vi "Save Macro.vi"(7 "Macro Name":string, 8 "error in (no error)":errorcluster, 10 "Macro Cluster":T1, 11 "refnum":T4) -> (0 "error out":errorcluster, 3 "refnum out":T4)   [LabVIEW 2023]
doc: "Saves <B>Macro Cluster</B> and its associated <B>Macro Name</B> to the config file defined by <B>refnum</B>."
uses:
  <vilib>/Utility/config.llb/Config Data RefNum.ctl
  CTLs/Macro Cluster V3.ctl
  CTLs/Step V3.ctl
  CTLs/Step Type V3.ctl
  <vilib>/Utility/config.llb/Write Key (String).vi
  <vilib>/Utility/config.llb/Write Key (I32).vi
  <vilib>/Utility/config.llb/NI_LVConfig.lvlib
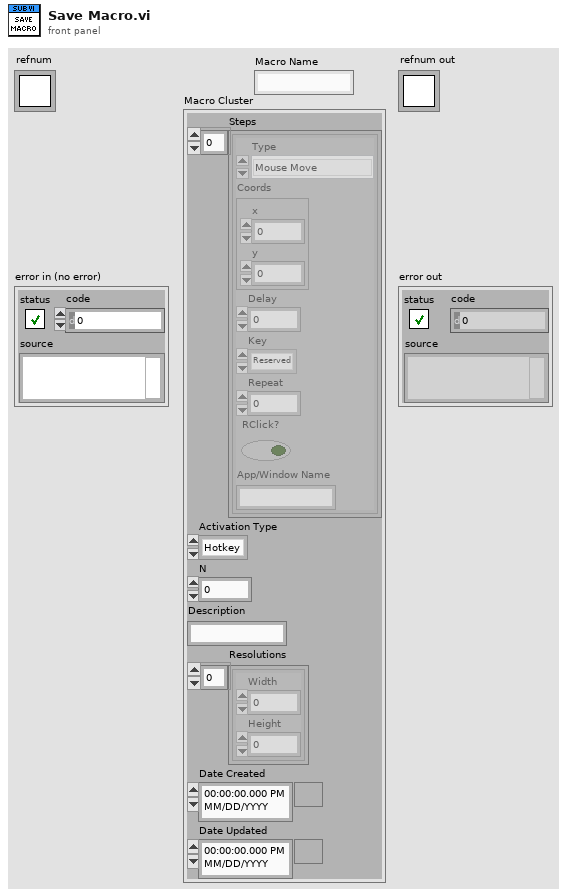
[diagram p1: front panel]
types:
  T1 = typedef "Macro Cluster V3.ctl" = cluster{"Steps":T2[], "Activation Type":enum32{"Hotkey", "Automatic"}, "N":i32, "Description":string, "Resolutions":cluster{"Width":i16, "Height":i16}[], "Date Created":timestamp, "Date Updated":timestamp}
  T2 = typedef "Step V3.ctl" = cluster{"Type":T3, "Coords":cluster{"x":i32, "y":i32}, "Delay":i32, "Key":u8, "Repeat":i32, "RClick?":bool, "App/Window Name":string}
  T3 = typedef "Step Type V3.ctl" = enum16{"Mouse Move", "Mouse Click", "Key Press", "Wait", "Mouse Down", "Mouse Up", "Key Down", "Key Up", "Run Application", "Quit Application", "Maximize Window", "Minimize Window", "Bring Window to Front", "Send Window to Back"}
  T4 = typedef "NI_LVConfig.lvlib/Config Data RefNum.ctl" = refnum<k1>
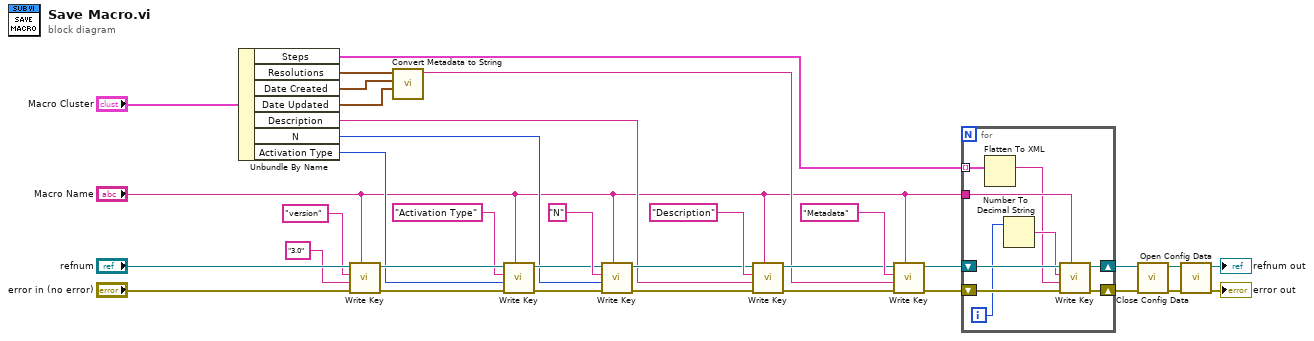
[diagram p0: block diagram]
diagram:
  n1 = Unbundle By Name("Macro Cluster") -> ("Steps"=w1:T2[], "Resolutions"=w10:cluster{"Width":i16, "Height":i16}[], "Date Created"=w9:timestamp, "Date Updated"=w8:timestamp, "Description"=w11:string, "N"=w12:i32, "Activation Type"=w13:enum32{"Hotkey", "Automatic"})
  n2 = call-poly <vilib>:"Write Key.vi"("section"="Macro Name", "error in (no error)"="error in (no error)", "value"="3.0" ("key"), "key"="version", "refnum"="refnum") -> ("error out"=w24:errorcluster, "refnum out"=w34:T4)  [unwired: 4 in, 1 out]
  n3 = call "Convert Metadata to String.vi"("Date Updated"=w8, "Date Created"=w9, "Resolutions"=w10) -> ("Metdata"=w7:string)  [unwired: 8 in]
  n4 = call-poly <vilib>:"Write Key.vi"("section"="Macro Name", "error in (no error)"=w24, "value"=w13, "key"="Activation Type", "refnum"=w34) -> ("error out"=w18:errorcluster, "refnum out"=w19:T4)  [unwired: 4 in, 1 out]
  n5 = call-poly <vilib>:"Write Key.vi"("section"="Macro Name", "error in (no error)"=w18, "value"=w12, "key"="N", "refnum"=w19) -> ("error out"=w16:errorcluster, "refnum out"=w17:T4)  [unwired: 4 in, 1 out]
  n6 = call-poly <vilib>:"Write Key.vi"("section"="Macro Name", "error in (no error)"=w16, "value"=w11, "key"="Description", "refnum"=w17) -> ("error out"=w14:errorcluster, "refnum out"=w15:T4)  [unwired: 4 in, 1 out]
  n7 = call-poly <vilib>:"Write Key.vi"("section"="Macro Name", "error in (no error)"=w14, "value"=w7, "key"="Metadata", "refnum"=w15) -> ("error out"=w6:errorcluster, "refnum out"=w5:T4)  [unwired: 4 in, 1 out]
  n8 = for {
    tunnel: "Macro Name" -> [w41]
    shift-right: [w39] -> w2
    shift-left: w6 -> [w43]
    shift-right: [w40] -> w3
    shift-left: w5 -> [w42]
    tunnel: w1 -> [w36] mode=indexing
    i -> [w37]
    n9 = Flatten To XML(6:w36) -> (2:w35:string)
    n10 = Number To Decimal String(number=w37) -> (decimal integer string=w38:string)  [unwired: 1 in]
    n11 = call-poly <vilib>:"Write Key.vi"("section"=w41, "error in (no error)"=w43, "value"=w35, "key"=w38, "refnum"=w42) -> ("error out"=w39:errorcluster, "refnum out"=w40:T4)  [unwired: 4 in, 1 out]
  }
  n12 = call <vilib>:"Close Config Data.vi"("error in (no error)"=w2, "refnum"=w3) -> ("error out"=w30:errorcluster, "file path"=w31:path)  [unwired: 8 in]
  n13 = call <vilib>:"Open Config Data.vi"("error in (no error)"=w30, "configuration file path"=w31) -> ("error out"=→"error out":errorcluster, "refnum"=→"refnum out":T4)  [unwired: 7 in, 1 out]
